vi "test2.vi"() -> ()   [LabVIEW 2020]
uses:
  <vilib>/Platform/TimedLoop/XDataNode/timing_clust.ctl
  <vilib>/Platform/TimedLoop/XDataNode/nitl_modes.ctl
  <vilib>/Platform/TimedLoop/XDataNode/wakeup.ctl
  70b06637-5d36-4187-b62a-e0680a00c2e7.vi
  <vilib>/platform/TimedLoop/XDataNode/XDataNode.xnode
  <vilib>/Platform/TimedLoop/XDataNode/XDNodeRunTimeDep.lvlib
panel:
  out "Stp2 Target Pos":dbl
  out "Stp1 Target Pos":dbl
  out "millisecond timer value 2":u32
  out "millisecond timer value":u32
  out "Stp2 Pos":dbl
  out "Stp1 Pos":dbl
  in  "Stp2 Speed":dbl
  in  "Stp1 Speed":dbl
  out "XY Graph 2":cluster{dbl[], dbl[]}[](graph)
  out "Moving":bool
  out "Tank":dbl(slide) scale=0.0..1.0
  out "Move Time":u32
  out "Distance":dbl
  out "Start Time":u32
  out "Start XY":cluster{"X":dbl, "Y":dbl}
  out "Draw Point XY":cluster{"X":dbl, "Y":dbl} {"X" format="%#.2f"; "Y" format="%#.2f"}
  in  "Clear History":bool
  out "Target XY":cluster{"X":dbl, "Y":dbl}
  out "Stopped":bool
  out "XY Graph":cluster{dbl[], dbl[]}[](graph)
  in  "Stop":bool
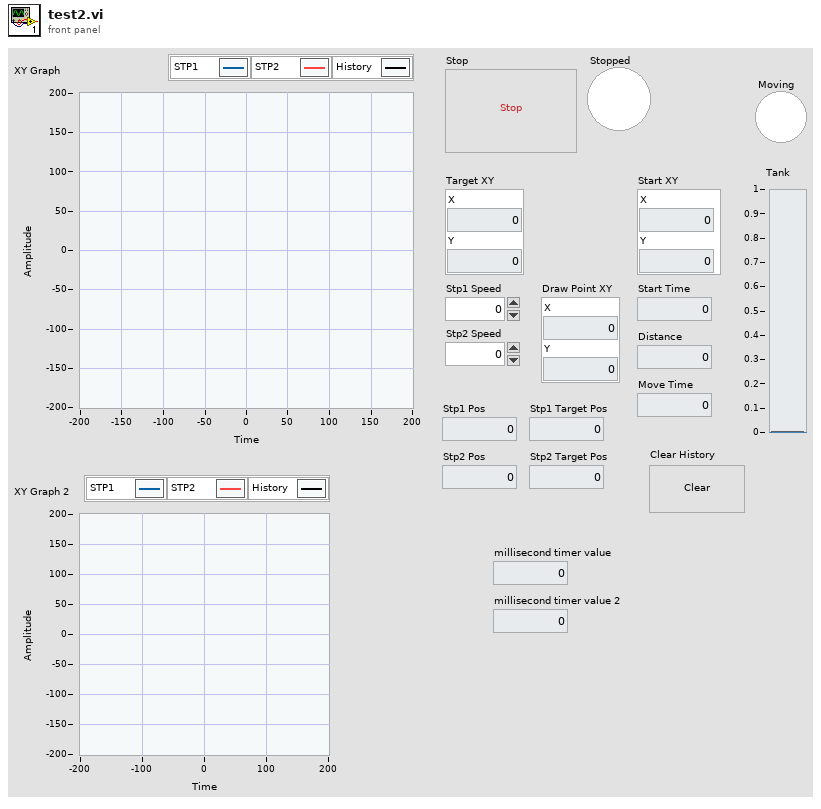
[diagram p1: front panel]
types:
  T1 = typedef "XDNodeRunTimeDep.lvlib/timing_clust.ctl" = cluster{"Expected End [f-1]":u64, "Actual End [f-1]":u64, "Finished Late? [f-1]":bool, "Expected End [i-1]":u64, "Actual End [i-1]":u64, "Finished Late? [i-1]":bool, "Expected Start [i]":u64, "Actual Start [i]":u64, "Expected Start [f]":u64, "Actual Start [f]":u64, "Source Name":string, "Structure Name":string, "Period":i64, "Deadline":i64, "Offset":i64, "Start":i64, "Priority":i32, "Timeout":i32, "Mode":T2, "Wakeup Reason":T3, "Error":errorcluster, "Source Type":string, "Secondary Source Type":string, "Global End Time":u64, "Global Start Time":u64, "Frame Duration":u64, "Iteration Duration":u64, "Assigned CPU":i32, "I/O Scan Engine Mode":u32}
  T2 = typedef "XDNodeRunTimeDep.lvlib/nitl_modes.ctl" = enum32{"No Change", "Process missed periods, maintain original phase", "Discard missed periods, maintain original phase", "Process missed periods, ignore original phase", "Discard missed periods, ignore original phase"}
  T3 = typedef "XDNodeRunTimeDep.lvlib/wakeup.ctl" = enum32{"Normal", "Aborted", "Asynchronous wakeup", "Timing source error", "Timed loop error", "Timeout"}
  T4 = typedef "LVPoint32TypeDef.ctl" = cluster{"Horizontal":i32, "Vertical":i32}
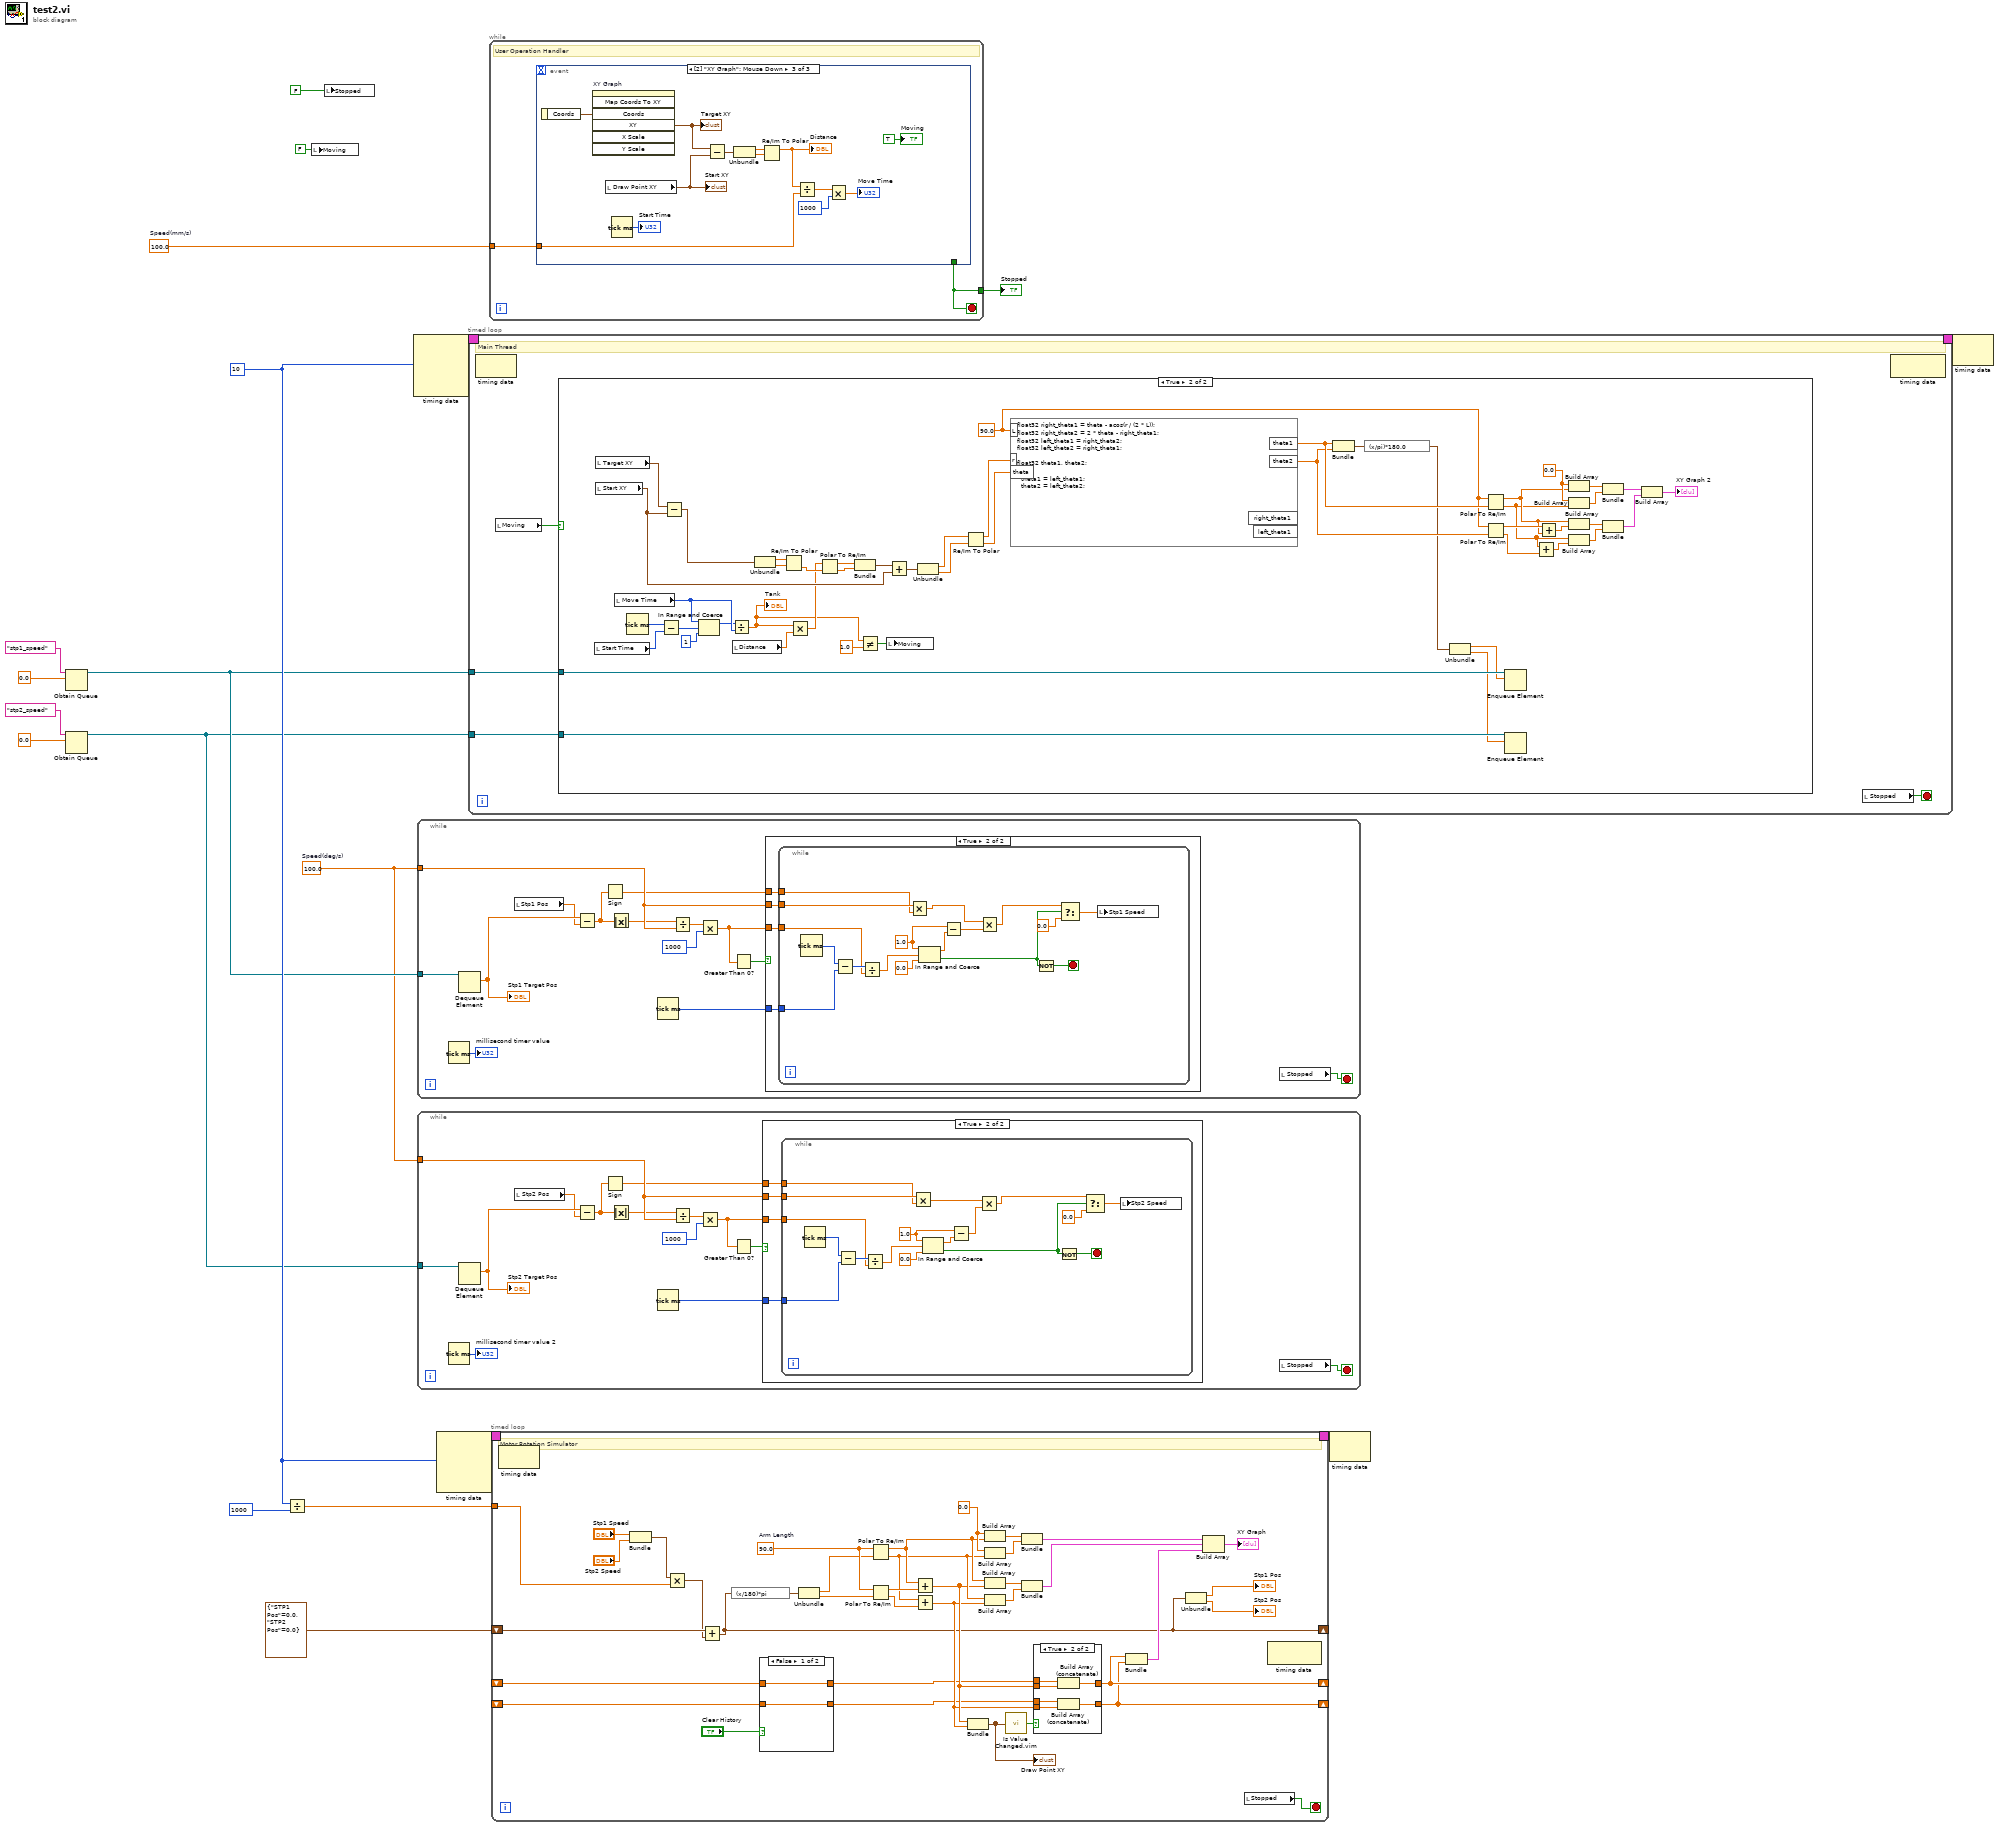
[diagram p0: block diagram]
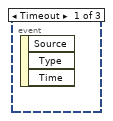
[diagram p7: hidden frame]
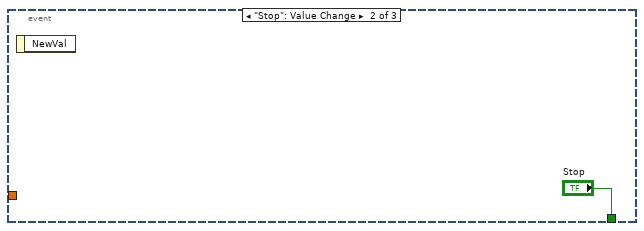
[diagram p8: hidden frame]
diagram:
  w4 = 100.0  # Speed(deg/s)
  w10 = 100.0  # Speed(mm/s)
  w8 = i64 10 ("Period")
  n1 = Obtain Queue(name (unnamed)="stp1_speed", element data type=0.0) -> (queue out=w6:refnum<queue>)  [unwired: 3 in, 2 out]
  n2 = Obtain Queue(name (unnamed)="stp2_speed", element data type=0.0) -> (queue out=w1:refnum<queue>)  [unwired: 3 in, 2 out]
  n3 = Divide(x=w8, y=i64 1000) -> (x/y=w11:dbl)
  n4 = local write "Moving"(FALSE ("Moving")) -> ()
  n5 = local write "Stopped"(FALSE ("Stopped")) -> ()
  n6 = node-c288(w8) -> (w16:T1)  [unwired: 3 in]
  n7 = while {
    tunnel: w6 -> [w33]
    tunnel: w4 -> [w27]
    stop <- w32 stop-if-true
    n8 = Tick Count (ms)() -> (millisecond timer value=→"millisecond timer value":u32)
    n9 = Dequeue Element(queue=w33) -> (element=w31:dbl)  [unwired: 2 in, 3 out]
    "Stp1 Target Pos" <- w31
    n10 = local read "Stp1 Pos"() -> (w23:dbl)
    n11 = Subtract(x=w31, y=w23) -> (x-y=w25:dbl)
    n12 = Sign(1:w25) -> (0:w24:dbl)
    n13 = Absolute Value(x=w25) -> (abs(x)=w26:dbl)
    n14 = Tick Count (ms)() -> (millisecond timer value=w28:u32)
    n15 = Divide(x=w26, y=w27) -> (x/y=w30:dbl)
    n16 = Multiply(x=w30, y=u32 1000 ("millisecond timer value")) -> (x*y=w21:dbl)
    n17 = Greater Than 0?(x=w21) -> (x > 0?=w20:bool)
    n18 = case shown="True" w20 {
      tunnel: w28 -> [_ w37]
      tunnel: w27 -> [_ w36]
      tunnel: w24 -> [_ w35]
      tunnel: w21 -> [_ w34]
      frame False {
      }
      frame True {
        n19 = while {
          tunnel: w34 -> [w53]
          tunnel: w37 -> [w49]
          tunnel: w36 -> [w45]
          tunnel: w35 -> [w44]
          stop <- w48 stop-if-true
          w41 = 1.0
          n20 = Tick Count (ms)() -> (millisecond timer value=w50:u32)
          n21 = Subtract(x=w50, y=w49) -> (x-y=w54:u32)
          n22 = Divide(x=w54, y=w53) -> (x/y=w52:dbl)
          n23 = Multiply(x=w45, y=w44) -> (x*y=w40:dbl)
          n24 = In Range and Coerce(upper limit=w41, x=w52, lower limit=0.0) -> (coerced(x)=w42:dbl, In Range?=w47:bool)
          n25 = Subtract(x=w41, y=w42) -> (x-y=w39:dbl)
          n26 = Multiply(x=w40, y=w39) -> (x*y=w38:dbl)
          n27 = Not(x=w47) -> (.not. x?=w48:bool)
          n28 = Select(t=w38, s=w47, f=0.0) -> (s? t:f=w43:dbl)
          n29 = local write "Stp1 Speed"(w43) -> ()
        }
      }
    }
    n30 = local read "Stopped"() -> (w32:bool)
  }
  n31 = while {
    tunnel: w4 -> [w63]
    tunnel: w1 -> [w59]
    stop <- w68 stop-if-true
    n32 = Tick Count (ms)() -> (millisecond timer value=→"millisecond timer value 2":u32)
    n33 = Dequeue Element(queue=w59) -> (element=w67:dbl)  [unwired: 2 in, 3 out]
    "Stp2 Target Pos" <- w67
    n34 = local read "Stp2 Pos"() -> (w58:dbl)
    n35 = Subtract(x=w67, y=w58) -> (x-y=w61:dbl)
    n36 = Sign(1:w61) -> (0:w60:dbl)
    n37 = Absolute Value(x=w61) -> (abs(x)=w62:dbl)
    n38 = Tick Count (ms)() -> (millisecond timer value=w64:u32)
    n39 = Divide(x=w62, y=w63) -> (x/y=w66:dbl)
    n40 = Multiply(x=w66, y=u32 1000 ("millisecond timer value")) -> (x*y=w56:dbl)
    n41 = Greater Than 0?(x=w56) -> (x > 0?=w55:bool)
    n42 = case shown="True" w55 {
      tunnel: w64 -> [_ w72]
      tunnel: w63 -> [_ w71]
      tunnel: w60 -> [_ w70]
      tunnel: w56 -> [_ w69]
      frame False {
      }
      frame True {
        n43 = while {
          tunnel: w69 -> [w88]
          tunnel: w72 -> [w84]
          tunnel: w71 -> [w80]
          tunnel: w70 -> [w79]
          stop <- w83 stop-if-true
          w77 = 1.0
          n44 = Tick Count (ms)() -> (millisecond timer value=w85:u32)
          n45 = Subtract(x=w85, y=w84) -> (x-y=w89:u32)
          n46 = Divide(x=w89, y=w88) -> (x/y=w87:dbl)
          n47 = Multiply(x=w80, y=w79) -> (x*y=w75:dbl)
          n48 = In Range and Coerce(upper limit=w77, x=w87, lower limit=0.0) -> (coerced(x)=w76:dbl, In Range?=w82:bool)
          n49 = Subtract(x=w77, y=w76) -> (x-y=w74:dbl)
          n50 = Multiply(x=w75, y=w74) -> (x*y=w73:dbl)
          n51 = Not(x=w82) -> (.not. x?=w83:bool)
          n52 = Select(t=w73, s=w82, f=0.0) -> (s? t:f=w78:dbl)
          n53 = local write "Stp2 Speed"(w78) -> ()
        }
      }
    }
    n54 = local read "Stopped"() -> (w68:bool)
  }
  n55 = node-c288(w8) -> (w19:T1)  [unwired: 3 in]
  n56 = timed-loop {
    timing: w16 -> [_]
    timing-out: [_] -> w15
    tunnel: w6 -> [w91]
    tunnel: w1 -> [w90]
    stop <- w93 stop-if-true
    # "Main Thread"
    n57 = node-c288() -> ()  [unwired: 1 in, 1 out]
    n58 = local read "Moving"() -> (w92:bool)
    n59 = case shown="True" w92 {
      tunnel: w91 -> [_ w117]
      tunnel: w90 -> [_ w96]
      frame False {
      }
      frame True {
        w113 = 0.0 ("element")
        w114 = 90.0 ("input variable")
        n60 = local read "Start Time"() -> (w140:u32)
        n61 = local read "Target XY"() -> (w99:cluster{"X":dbl, "Y":dbl})
        n62 = local read "Start XY"() -> (w131:cluster{"X":dbl, "Y":dbl})
        n63 = local read "Move Time"() -> (w126:u32)
        n64 = Tick Count (ms)() -> (millisecond timer value=w141:u32)
        n65 = Subtract(x=w141, y=w140) -> (x-y=w127:u32)
        n66 = Subtract(x=w99, y=w131) -> (x-y=w138:cluster{"X":dbl, "Y":dbl})
        n67 = In Range and Coerce(upper limit=w126, x=w127, lower limit=u32 1) -> (coerced(x)=w124:u32)  [unwired: 1 out]
        n68 = Divide(x=w124, y=w126) -> (x/y=w120:dbl)
        "Tank" <- w120
        n69 = local read "Distance"() -> (w139:dbl)
        n70 = Unbundle(w138) -> ("X"=w137:dbl, "Y"=w136:dbl)
        n71 = Re/Im To Polar(2:w136, 3:w137) -> (0:w135:dbl)  [unwired: 1 out]
        n72 = Multiply(x=w120, y=w139) -> (x*y=w123:dbl)
        n73 = Polar To Re/Im(2:w135, 3:w123) -> (0:w133:dbl, 1:w134:dbl)
        n74 = Bundle(w134, w133) -> (w132:cluster{dbl, dbl})  [unwired: 1 in]
        n75 = Not Equal?(x=w120, y=1.0) -> (x != y?=w118:bool)
        n76 = local write "Moving"(w118) -> ()
        n77 = Add(x=w132, y=w131) -> (x+y=w94:cluster{dbl, dbl})
        n78 = Unbundle(w94) -> (w130:dbl, w129:dbl)
        n79 = Re/Im To Polar(2:w129, 3:w130) -> (0:w128:dbl, 1:w122:dbl)
        n80 = formula code="float32 right_theta1 = theta - acos(r / (2 * L));\nfloat32 right_theta2 = 2 * theta - right_theta1;\nfloat32 left_theta1 = right_theta2;\nfloat32 left_theta2 = right_theta1;\n\nfloat32 theta1, theta2;\n\n  theta1 = left_theta1;\n  theta2 = left_theta2;"("r"=w122, "theta"=w128, "L"=w114) -> ("theta1"=w116:sgl, "theta2"=w115:sgl)  [unwired: 2 out]
        n81 = Bundle(w116, w115) -> (w121:cluster{sgl, sgl})  [unwired: 1 in]
        n82 = expression code="(x/pi)*180.0"(w121) -> (w98:cluster{sgl, sgl})
        n83 = Unbundle(w98) -> (w97:sgl, w95:sgl)
        n84 = Polar To Re/Im(2:w116, 3:w114) -> (0:w101:dbl, 1:w103:dbl)
        n85 = Polar To Re/Im(2:w115, 3:w114) -> (0:w102:dbl, 1:w105:dbl)
        n86 = Enqueue Element(queue=w117, element=w97) -> ()  [unwired: 2 in, 3 out]
        n87 = Enqueue Element(queue=w96, element=w95) -> ()  [unwired: 2 in, 3 out]
        n88 = Add(x=w101, y=w102) -> (x+y=w100:dbl)
        n89 = Add(x=w105, y=w103) -> (x+y=w104:dbl)
        n90 = Build Array(w113, w103) -> (w112:dbl[])
        n91 = Build Array(w113, w101) -> (w111:dbl[])
        n92 = Build Array(w103, w104) -> (w110:dbl[])
        n93 = Build Array(w101, w100) -> (w109:dbl[])
        n94 = Bundle(w112, w111) -> (w108:cluster{dbl[], dbl[]})  [unwired: 1 in]
        n95 = Bundle(w110, w109) -> (w107:cluster{dbl[], dbl[]})  [unwired: 1 in]
        n96 = Build Array(w108, w107) -> (→"XY Graph 2":cluster{dbl[], dbl[]}[])
      }
    }
    n97 = local read "Stopped"() -> (w93:bool)
    n98 = node-c288() -> ()  [unwired: 1 in, 1 out]
  }
  n99 = while {
    tunnel: [w145] -> w14
    tunnel: w10 -> [w144]
    stop <- w145 stop-if-true
    # "User Operation Handler"
    n100 = event shown="[2] \"XY Graph\": Mouse Down" {
      selector: _ -> [_ _ _]
      dyn-events: _ -> [_ _ _]
      timeout: _ -> [_ _ _]
      tunnel: [_ "Stop" _] -> w145
      tunnel: w144 -> [_ _ w151]
      event Timeout {
        n101 = event-data() -> ()  [unwired: 1 in, 3 out]
      }
      event "Stop": Value Change {
        n102 = event-data() -> ()  [unwired: 1 in, 1 out]
      }
      event "XY Graph": Mouse Down {
        n103 = event-data() -> ("Coords"=w159:T4)  [unwired: 1 in]
        n104 = invoke on="XY Graph" class="XYGraph (strict)" method="Map Coords To XY"("Coords"=w159) -> ("XY"=w157:cluster{"X":dbl, "Y":dbl})  [unwired: 6 in, 6 out]
        "Target XY" <- w157
        n105 = local read "Draw Point XY"() -> (w156:cluster{"X":dbl, "Y":dbl})
        "Start XY" <- w156
        n106 = Tick Count (ms)() -> (millisecond timer value=→"Start Time":u32)
        n107 = Subtract(x=w157, y=w156) -> (x-y=w155:cluster{"X":dbl, "Y":dbl})
        n108 = Unbundle(w155) -> ("X"=w154:dbl, "Y"=w153:dbl)
        n109 = Re/Im To Polar(2:w153, 3:w154) -> (1:w152:dbl)  [unwired: 1 out]
        "Distance" <- w152
        n110 = Divide(x=w152, y=w151) -> (x/y=w150:dbl)
        n111 = Multiply(x=w150, y=u32 1000 ("millisecond timer value")) -> (x*y=→"Move Time":dbl)
        "Moving" <- TRUE ("Moving")
      }
    }
  }
  "Stopped" <- w14
  n112 = timed-loop {
    timing: w19 -> [_]
    timing-out: [_] -> w18
    shift-right: [w162] -> _
    shift-left: cluster{"STP1 Pos":dbl, "STP2 Pos":dbl} {"STP1 Pos"=0.0, "STP2 Pos"=0.0} -> [w194]
    shift-right: [w176] -> _
    shift-left: _ -> [w172]
    shift-right: [w175] -> _
    shift-left: _ -> [w170]
    tunnel: w11 -> [w167]
    stop <- w197 stop-if-true
    w185 = 0.0 ("element")
    w193 = 90.0  # Arm Length
    # "Motor Rotation Simulator"
    n113 = node-c288() -> ()  [unwired: 1 in, 1 out]
    n114 = Bundle("Stp1 Speed"="Stp1 Speed", "Stp2 Speed"="Stp2 Speed") -> (w163:cluster{"Stp1 Speed":dbl, "Stp2 Speed":dbl})  [unwired: 1 in]
    n115 = Multiply(x=w163, y=w167) -> (x*y=w168:cluster{"Stp1 Speed":dbl, "Stp2 Speed":dbl})
    n116 = Add(x=w194, y=w168) -> (x+y=w162:cluster{dbl, dbl})
    n117 = expression code="(x/180)*pi"(w162) -> (w192:cluster{dbl, dbl})
    n118 = case shown="False" "Clear History" {
      tunnel: [w199 _] -> w173
      tunnel: w172 -> [w199 _]
      tunnel: [w198 _] -> w171
      tunnel: w170 -> [w198 _]
      frame False {
      }
      frame True {
      }
    }
    n119 = Unbundle(w192) -> (w191:dbl, w190:dbl)
    n120 = Polar To Re/Im(2:w191, 3:w193) -> (0:w180:dbl, 1:w181:dbl)
    n121 = Polar To Re/Im(2:w190, 3:w193) -> (0:w188:dbl, 1:w189:dbl)
    n122 = Add(x=w181, y=w189) -> (x+y=w179:dbl)
    n123 = Add(x=w180, y=w188) -> (x+y=w178:dbl)
    n124 = Bundle(w179, w178) -> (w166:cluster{dbl, dbl})  [unwired: 1 in]
    "Draw Point XY" <- w166
    n125 = Build Array(w185, w181) -> (w196:dbl[])
    n126 = Build Array(w185, w180) -> (w195:dbl[])
    n127 = Build Array(w181, w179) -> (w186:dbl[])
    n128 = Build Array(w180, w178) -> (w187:dbl[])
    n129 = call "Is Value Changed.vim"("value"=w166) -> ("changed or first call?"=w177:bool)
    n130 = Bundle(w196, w195) -> (w184:cluster{dbl[], dbl[]})  [unwired: 1 in]
    n131 = Bundle(w186, w187) -> (w183:cluster{dbl[], dbl[]})  [unwired: 1 in]
    n132 = case shown="True" w177 {
      tunnel: w179 -> [_ w207]
      tunnel: w178 -> [_ w206]
      tunnel: [w201 w205] -> w176
      tunnel: [w200 w204] -> w175
      tunnel: w173 -> [w201 w203]
      tunnel: w171 -> [w200 w202]
      frame False {
      }
      frame True {
        n133 = Build Array (concatenate)(w203, w207) -> (w205:dbl[])
        n134 = Build Array (concatenate)(w202, w206) -> (w204:dbl[])
      }
    }
    n135 = Bundle(w176, w175) -> (w174:cluster{dbl[], dbl[]})  [unwired: 1 in]
    n136 = Unbundle(w162) -> (→"Stp1 Pos":dbl, →"Stp2 Pos":dbl)
    n137 = Build Array(w184, w183, w174) -> (→"XY Graph":cluster{dbl[], dbl[]}[])
    n138 = local read "Stopped"() -> (w197:bool)
    n139 = node-c288() -> ()  [unwired: 1 in, 1 out]
  }
  n140 = node-c288(w18) -> ()  [unwired: 1 out]
  n141 = node-c288(w15) -> ()  [unwired: 1 out]
